vi "Funct TIFF export-Generate image from data.vi"(4 "Horisontal (T)":bool=TRUE, 6 "3D":u16[][](array[numeric]), 8 "error in (no error)":errorcluster, 9 "Rectangle index":i32, 10 "Image Name":string, 11 "Refnum in":T1) -> (0 "error out":errorcluster, 3 "Refnum out":T1)   [LabVIEW 2017]
uses:
  <vilib>/vision/Image Controls.llb/IMAQ Image.ctl
  <vilib>/vision/NI_Vision_Development_Module.lvlib
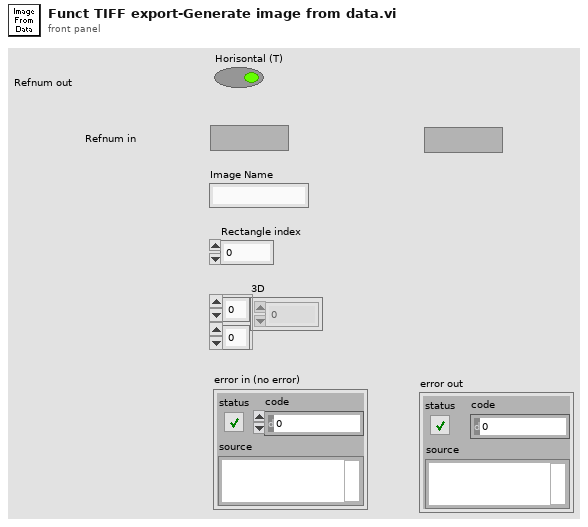
[diagram p1: front panel]
types:
  T1 = typedef "IMAQ Image.ctl" = refnum<image>
  T2 = typedef "Image Type" = u32
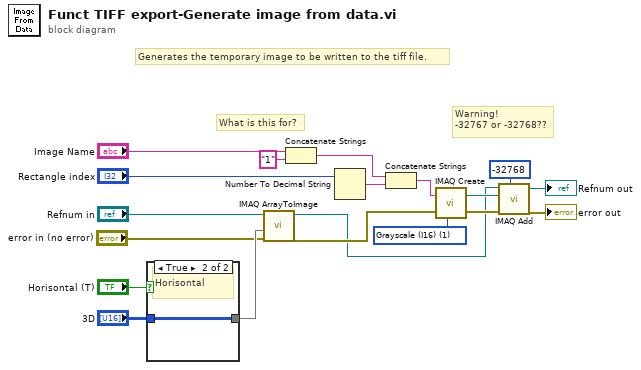
[diagram p0: block diagram]
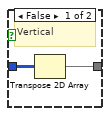
[diagram p2: hidden frame]
diagram:
  w18 = T2 1 items=["Grayscale (U8)", "Grayscale (I16)", "Grayscale (SGL)", "Complex (CSG)", "RGB (U32)", "HSL (U32)", "RGB (U64)"] ("Image Type")
  # "Generates the temporary image to be written to the tiff file."
  # "Warning!\n-32767 or -32768??"
  # "What is this for?"
  n1 = case shown="True" "Horisontal (T)" {
    tunnel: "3D" -> [w21 w22]
    tunnel: [w20 w22] -> w12
    frame False {
      # "Vertical"
      n2 = Transpose 2D Array(2D array=w21) -> (transposed array=w20:u16[][])
    }
    frame True {
      # "Horisontal"
    }
  }
  n3 = call "IMAQ ArrayToImage"("error in (no error)"="error in (no error)", "Image Pixels (I16)"=w12, "Image"="Refnum in") -> ("error out"=w13:errorcluster, "Image Out"=w3:T1)  [unwired: 7 in]
  n4 = Concatenate Strings("Image Name", "1" ("string")) -> (w10:string)
  n5 = Number To Decimal String(number="Rectangle index") -> (decimal integer string=w17:string)  [unwired: 1 in]
  n6 = Concatenate Strings(w10, w17) -> (w16:string)
  n7 = call "IMAQ Create"("Image Name"=w16, "Image Type"=w18, "error in (no error)"=w13) -> ("New Image"=w15:T1, "error out"=w14:errorcluster)  [unwired: 2 in]
  n8 = call "IMAQ Add"("Image Src A"=w3, "Constant"=i16 -32768, "Image Dst"=w15, "error in (no error)"=w14) -> ("Image Dst Out"=→"Refnum out":T1, "error out"=→"error out":errorcluster)  [unwired: 3 in]
